vi "AddSubExperiment.vi"(8 "error in (no error)":errorcluster, 10 "channel":u8, 11 "deviceName":string) -> (0 "error out":errorcluster)   [LabVIEW 2018]
doc: "EXPORT void AisAddSubExperiment(const char* deviceName, uint8_t channel);"
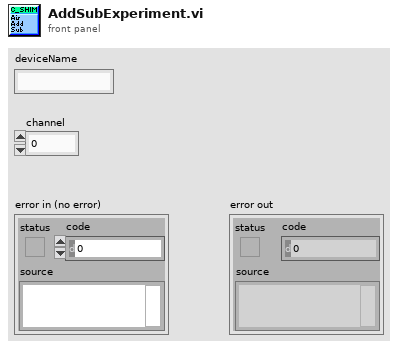
[diagram p1: front panel]
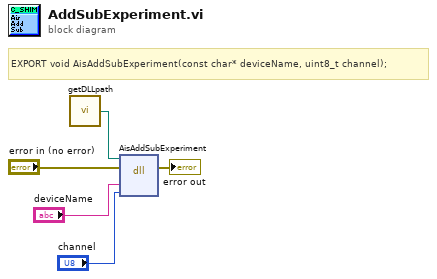
[diagram p0: block diagram]
diagram:
  # "EXPORT void AisAddSubExperiment(const char* deviceName, uint8_t channel);"
  n1 = call "getDLLpath.vi"() -> ("DLL_Path"=w1:path)
  n2 = dll-call lib="?" fn="AisAddSubExperiment"(path in=w1, error in="error in (no error)", "deviceName"="deviceName", "channel"="channel") -> (error out=→"error out":errorcluster)  [unwired: 4 in, 1 out]
